vi "setFont.vi"(8 "error in (no error)":errorcluster, 10 "Font":T1={"Name"="Calibri", "Size"=12, "Bold"=FALSE, "Italic"=FALSE, "Underline"=18, "Strike"=FALSE, "Color"=0} {"Underline" items=["Single"=1, "Words"=2, "Double"=3, "Thick"=4, "Dotted"=5, "DottedHeavy"=6, "Dash"=7, "DashedHeavy"=8, "DashLong"=9, "DashLongHeavy"=10, "DotDash"=11, "DashDotHeavy"=12, "DotDotDash"=13, "DashDotDotHeavy"=14, "Wave"=15, "WavyHeavy"=16, "WavyDouble"=17, "None"=18]}, 11 "Font in":refnum<class "Font.lvclass">) -> (0 "error out":errorcluster, 3 "Font out":refnum<class "Font.lvclass">)   [LabVIEW 2020, in "Fonts.lvlib" / "Font.lvclass"]
uses:
  Font.lvclass
  Font--cluster.ctl
  Underline--ring.ctl
  Font.lvclass/Font.ctl
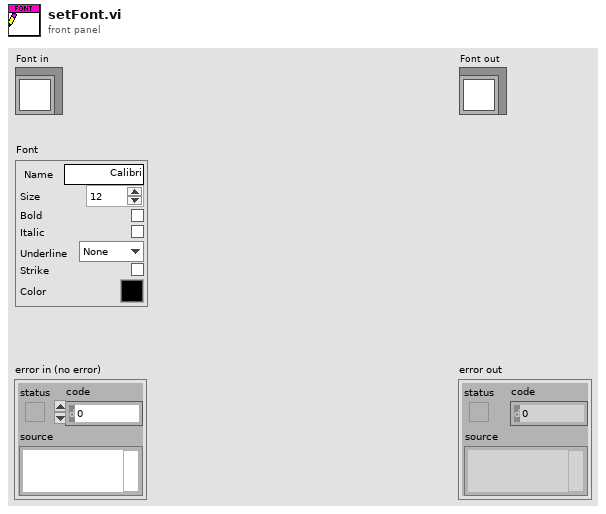
[diagram p1: front panel]
types:
  T1 = typedef "Fonts.lvlib/Font.lvclass/Font--cluster.ctl" = cluster{"Name":string, "Size":i32, "Bold":bool, "Italic":bool, "Underline":T2, "Strike":bool, "Color":u32}
  T2 = typedef "Fonts.lvlib/Font.lvclass/Underline--ring.ctl" = i32
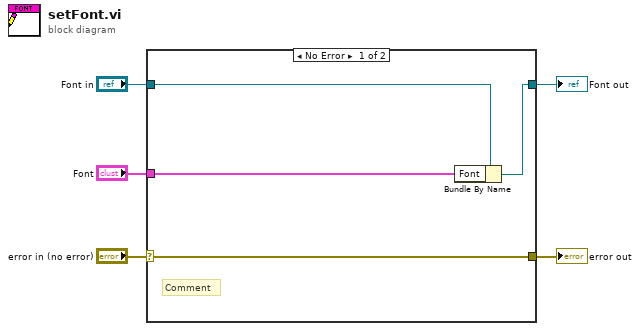
[diagram p0: block diagram]
diagram:
  n1 = case shown="No Error" "error in (no error)" {
    selector: "error in (no error)" -> [w9 w10]
    tunnel: [w9 w10] -> w4
    tunnel: [w7 w11] -> w2
    tunnel: "Font in" -> [w8 w11]
    tunnel: "Font" -> [w6 _]
    frame No Error {
      # "Comment"
      n2 = Bundle By Name(cluster=w8, "Font"=w6) -> (w7:refnum<class "Font.lvclass">)
    }
    frame Error {
    }
  }
  "error out" <- w4
  "Font out" <- w2
